vi "why_jiggle.vi"() -> ()   [LabVIEW 2023]
uses:
  Supporting VIs/Sampling frequency.ctl
  Arun_test/Control 1.ctl
  Supporting VIs/Logic states.ctl
  Supporting VIs/Motor states.ctl
  Supporting VIs/Queue names.ctl
  <instrlib>/Arcus Driver 3.0.0/ArcusUsbComm/classes/Controller/_Controller.lvclass
  <instrlib>/Arcus Driver 3.0.0/ArcusUsbComm/common/controls/linear_direction.ctl
  Supporting VIs/Axes indices.ctl
  <vilib>/DAQmx/read.llb/DAQmx Read (Analog 1D DBL NChan 1Samp).vi
  <vilib>/Analysis/baseanly.llb/Vector x A.vi
  <vilib>/Analysis/baseanly.llb/A x Vector.vi
  <vilib>/DAQmx/create/channels.llb/DAQmx Create Channel (AI-Voltage-Basic).vi
  <vilib>/DAQmx/configure/timing.llb/DAQmx Timing (Sample Clock).vi
  <vilib>/DAQmx/miscellaneous.llb/DAQmx Fill In Error Info.vi
  <vilib>/Utility/file.llb/Write Delimited Spreadsheet (string).vi
  <vilib>/addons/control/pid/pid.llb/PID (DBL).vi
  <vilib>/Utility/file.llb/Write Delimited Spreadsheet (DBL).vi
  <vilib>/Analysis/NI_AALBase.lvlib
  <instrlib>/Arcus Driver 3.0.0/ArcusUsbComm/libraries/common.lvlib
  <vilib>/addons/control/pid/NI_PID_pid.lvlib
panel:
  in  "Wait [min]":dbl=30.0 format="%.2g"
  in  "Wait ?":bool=TRUE
  in  "Save file name":path=path "C:/Users/Egberts/Desktop/Tribometer/August 2020 Measurements/Tribometer/Late August 2020/test.txt"
  out "Apprx. Min Left":i32
  out "Cycles left":i32
  out "Test Progress":i32(slide) scale=0.0..5999.0
  in  "PID gains":T1={"proportional gain (Kc)"=0.02, "integral time (Ti, min)"=0.1, "derivative time (Td, min)"=0.001} {"derivative time (Td, min)" format="%.3f"; "integral time (Ti, min)" format="%.3f"; "proportional gain (Kc)" format="%.3f"}
  in  "output range":cluster{"output high":dbl, "output low":dbl}={"output high"=2.0, "output low"=-2.0} {"output low" format="%.2f"; "output high" format="%.2f"}
  out "x-position":i32
  out "z-position":string
  in  "set zero":bool
  out "Correction loop":i32
  out "received P":i32
  out "Actual Load":dbl
  out "Correction [N]":dbl format="%.2f"
  out "correction [p]":dbl
  out "to PID":i32
  out "dt out (s)":dbl=0.25 format="%.3f"
  in  "Testing Load [N]":dbl=20.0
  in  "Wear cycles":i32=3000
  in  "Track length [mm]":i32=15
  in  "x-Velocity [mm/s]":i32=6
  out "Manual control":bool
  in  "Approach":bool
  in  "DAQmx Device Name":tag="Dev1"
  in  "Out":bool
  in  "In":bool
  in  "Left":bool
  in  "Right":bool
  in  "Up":bool
  out "Estimated friction coefficient":dbl(graph)=-0.11599973982411911
  out "Smooth x":dbl(graph)=-1.1532615270996815
  out "Smooth z":dbl(graph)=9.94193201509139
  out "Dequeued Data":dbl[](graph)=[9.378691263157721, 10.717600289594278, 8.438969804942502, 9.318124790458075, 8.681089909963866, 9.970529667476073, 10.834102440336615, 9.183821958337319, 9.334582664259113, 9.226213467034226, 10.238553338370796, 11.173780758664948, 8.690449558950064, 9.261606371512476, 8.790570665988898, 9.887706352746802, 11.038667014275244, 8.916330650848511, 9.104119720861869, 8.923720573303449]
  out "Fixed amplitude Load":T2=8.923720573303449
  in  "ABORT":bool
  in  "Down":bool
  out "Aborted":bool
  out "Mean z":dbl[](array[numeric])
  out "Current reading":dbl[](array[numeric])
  in  "Averaging Level":i32=12
  out "Mean x":dbl[](array[numeric])
  out "Completed":bool
  out "Testing":bool
  out "Approaching":bool
  in  "TARE":bool
  in  "Sampling frequency (rate)":T3=100 items=["1000 Hz"=1000, " 500 Hz"=500, " 250 Hz"=250, "100 Hz"=100, "50 Hz"=50, "10 Hz"=10, "1 Hz"=1]
  in  "Calibration file":path=path "C:/Users/Egberts/Desktop/ATI Industrial Automation/FT21774.cal"
  # "Originally used to measure \nthe amount of positions needed\nto perform fast approach"
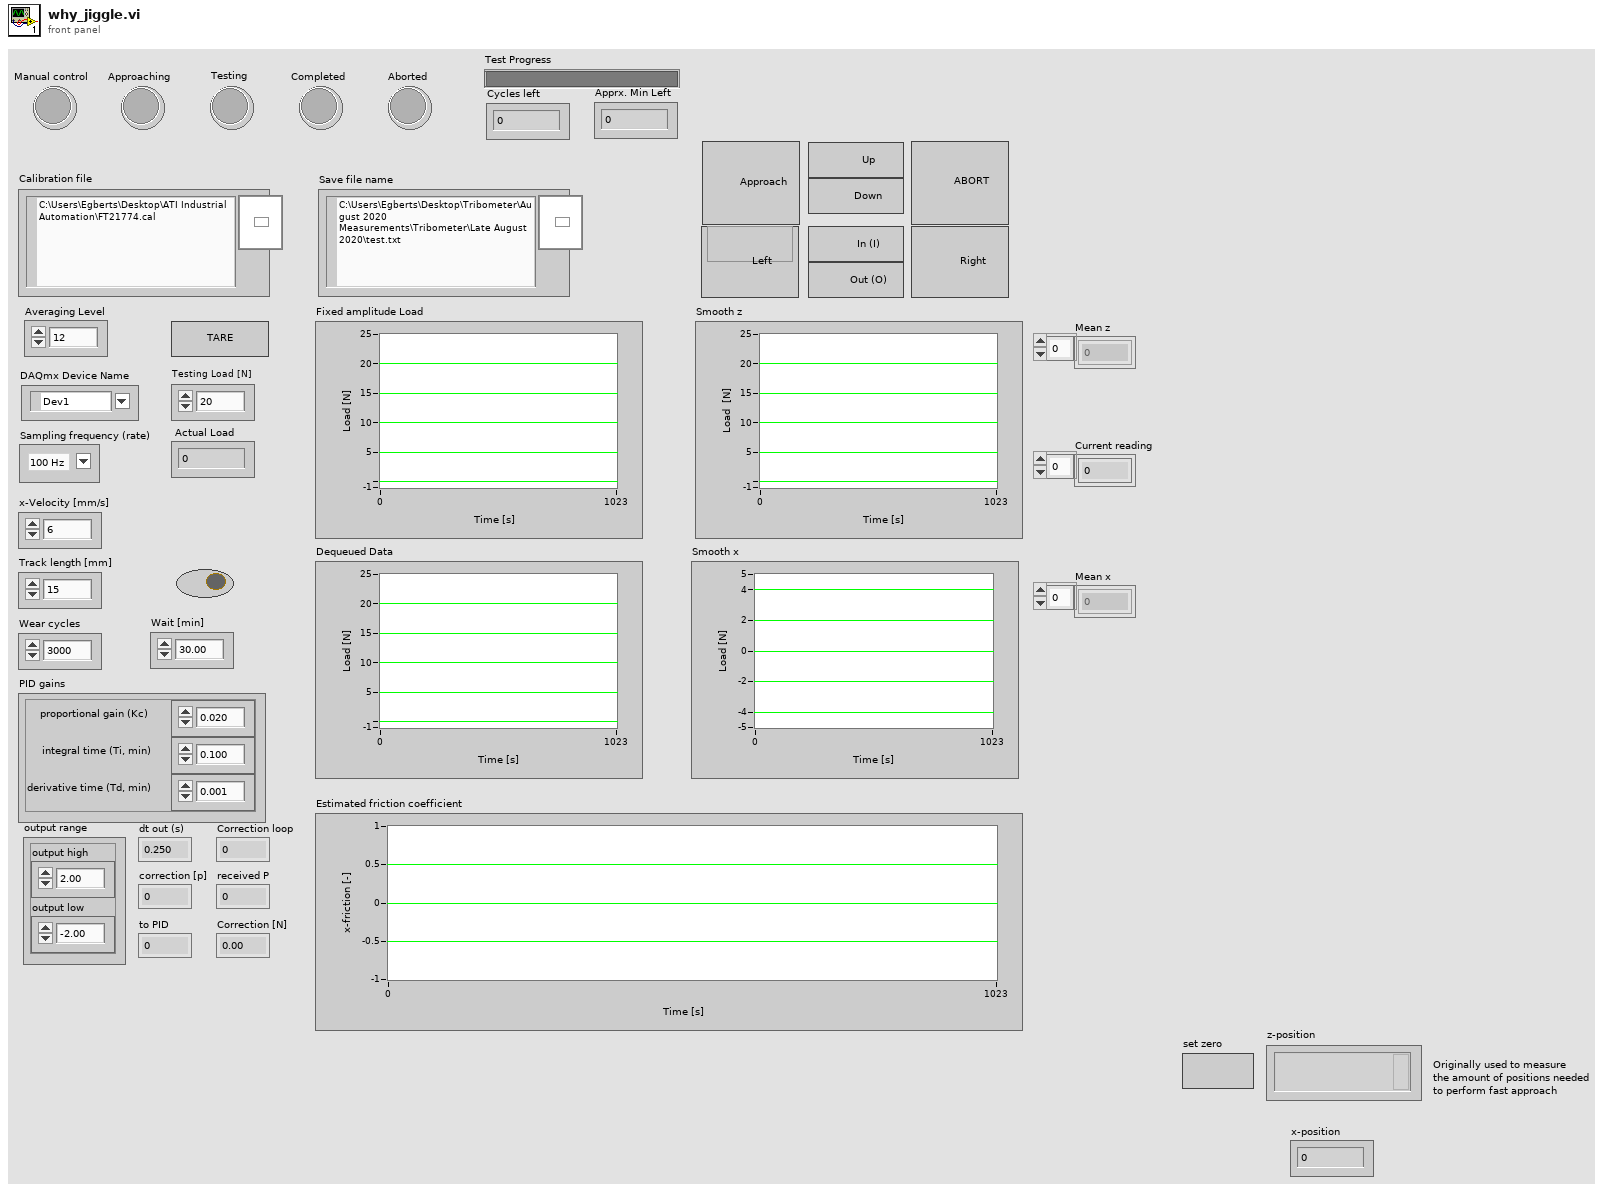
[diagram p1: front panel]
types:
  T1 = cluster{"proportional gain (Kc)":dbl, "integral time (Ti, min)":dbl, "derivative time (Td, min)":dbl}
  T2 = typedef "Control 1.ctl" = dbl
  T3 = typedef "Sampling frequency.ctl" = u16
  T4 = typedef "Queue names.ctl" = enum16{"Cell queue name", "z-axis ref queue", "x-axis ref queue", "tangent-axis ref queue", "y-axis ref queue", "to PID", "Feedback"}
  T5 = typedef "Motor states.ctl" = enum16{"Initialize", "Manual control", "Approaching", "Testing", "Terminate"}
  T6 = typedef "Logic states.ctl" = enum16{"Initialize", "Process", "Terminate"}
  T7 = enum8{"Enabled", "Disabled", "Disabled and Grayed Out"}
  T8 = cluster{"queue out":refnum<queue>, "error out":errorcluster}
  T9 = cluster{"task out":refnum<k21>, "error out":errorcluster}
  T10 = cluster{"reference (out)":refnum<class "_Controller.lvclass">, "error out":errorcluster}
  T11 = typedef "Axes indices.ctl" = enum16{"y-axis", "x-axis", "z-axis"}
  T12 = cluster{"queue out":refnum<queue>, "queue out":refnum<queue>, "queue out":refnum<queue>}
  T13 = typedef "common.lvlib/linear_direction.ctl" = enum16{"POS (+)", "NEG (-)"}
  T14 = typedef "lveventtype.ctl" = enum32{"Null", "Timeout", "Annotation Menu Selection", "Annotation Menu Selection?", "App Instance Close", "App Instance Close?", "Autoscale Range Change", "Bookmark Info Change", "Cell Edit", "Cell Edit?", "Cursor Grab", "Cursor Grab?", "Cursor Menu Selection", "Cursor Menu Selection?", "Cursor Move", "Cursor Release", "Data Change", "Direction Change", "Display State Change", "Drag Ended", "Drag Enter", "Drag Leave", "Drag Over", "Drag Source Update", "Drag Starting", "Drag Starting?", "Drop", "Exec State Change", "Key Down", "Key Down?", "Key Repeat", "Key Repeat?", "Key Up", "Listbox Double Click", "Menu Activation?", "Menu Selection (App)", "Menu Selection? (App)", "Menu Selection (User)", "Mouse Down", "Mouse Down?", "Mouse Enter", "Mouse Leave", "Mouse Move", "Mouse Up", "Mouse Wheel", "NI Security User Change (App)", "Pane Size", "Panel Close", "Panel Close?", "Panel Resize", "Plot Attribute Change", "Scale Range Change", "Shortcut Menu Activation?", "Shortcut Menu Selection (App)", "Shortcut Menu Selection? (App)", "Shortcut Menu Selection (User)", "Tree Double Click", "Tree Drag", "Tree Drag?", "Tree Drop", "Tree Drop?", "Tree Item Close", "Tree Item Close?", "Tree Item Open", "Tree Item Open?", "User Event", "Value Change"}
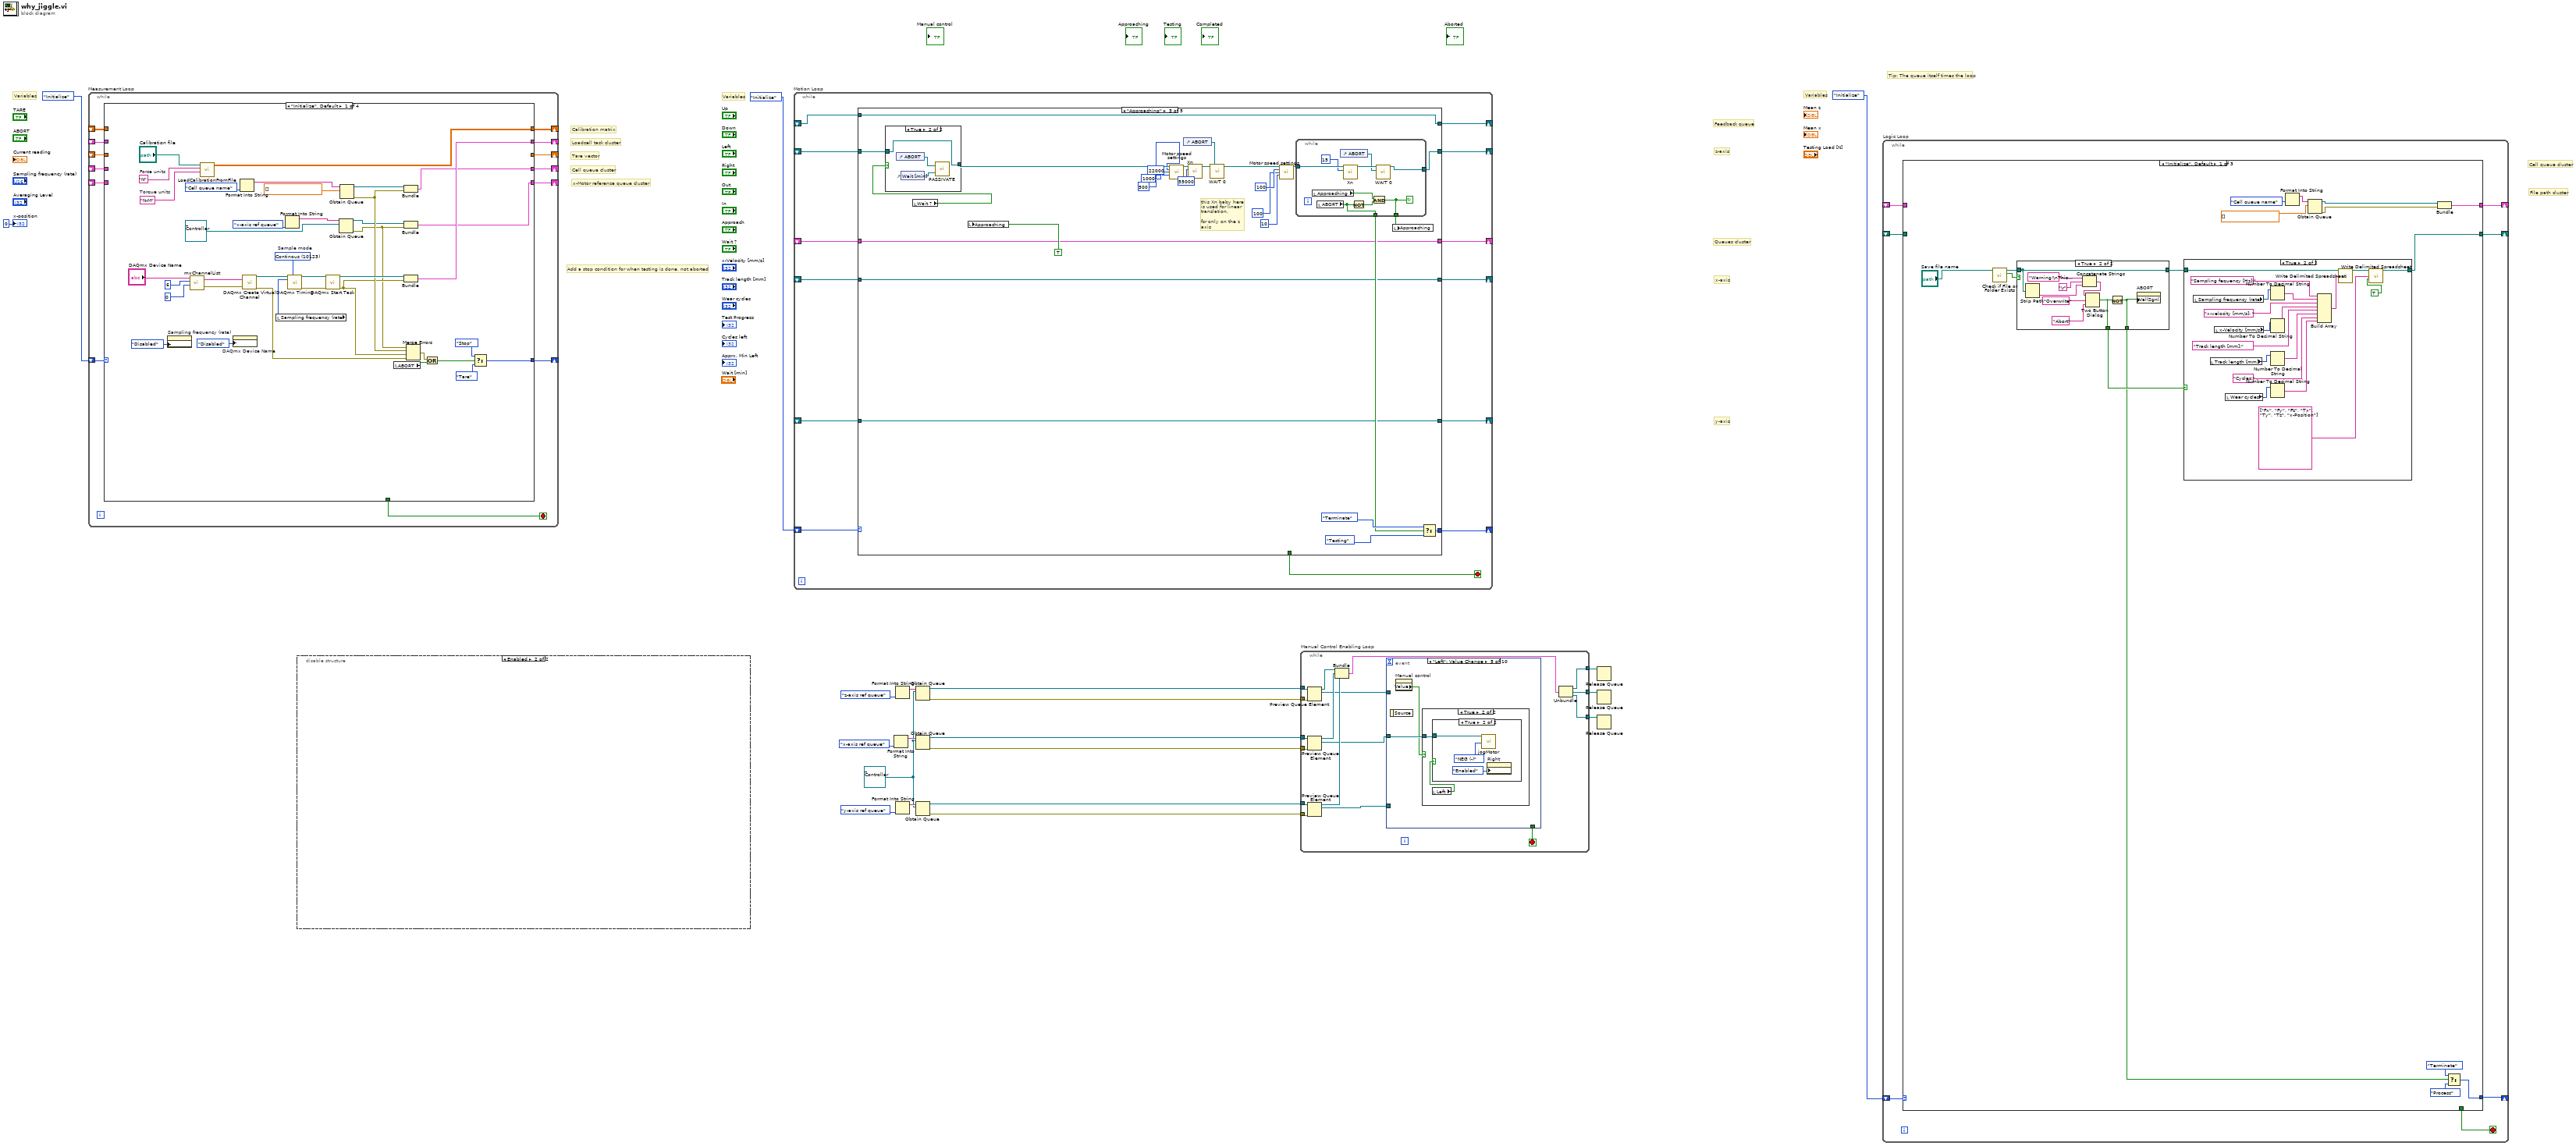
[diagram p0: block diagram]
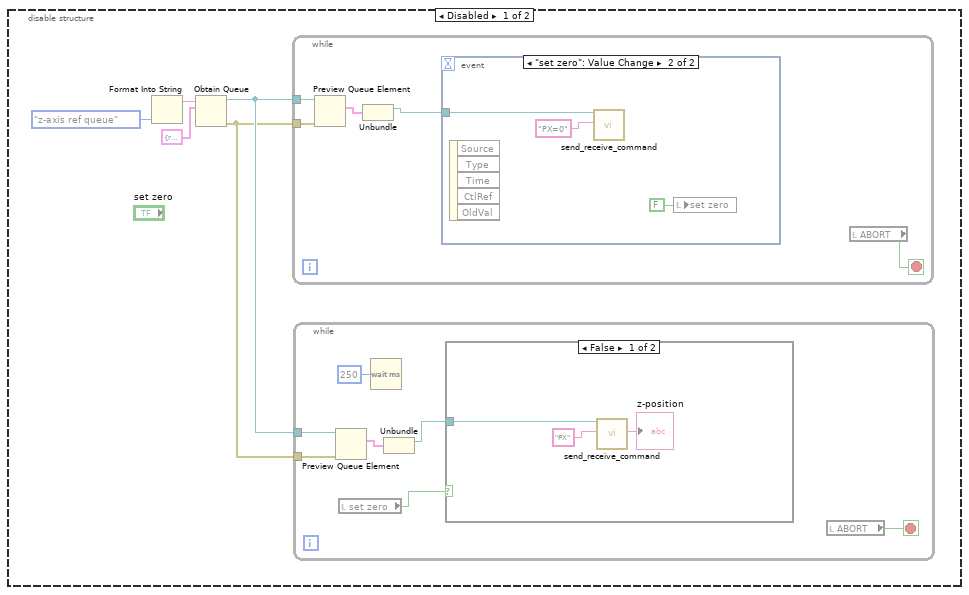
[diagram p2: hidden frame]
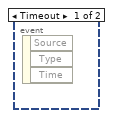
[diagram p4: hidden frame]
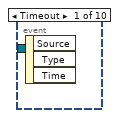
[diagram p5: hidden frame]
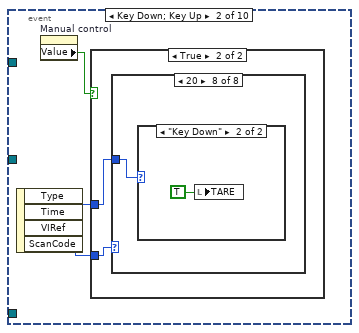
[diagram p6: hidden frame]
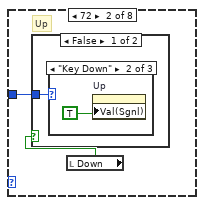
[diagram p9: hidden frame]
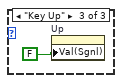
[diagram p11: hidden frame]
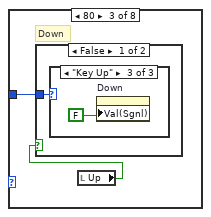
[diagram p13: hidden frame]
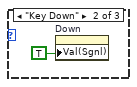
[diagram p15: hidden frame]
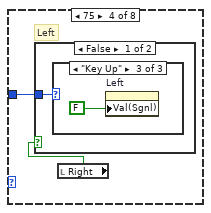
[diagram p17: hidden frame]
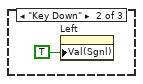
[diagram p19: hidden frame]
diagram:
  w1 = refnum<class "_Controller.lvclass"> refnum ("Controller in")
  # "Feedback queue"
  # "Queues cluster"
  # "x-Motor reference queue cluster"
  # "Add a stop condition for when testing is done, not aborted"
  # "y-axis"
  # "x-axis"
  # "z-axis"
  # "Variables"
  # "Variables"
  # "File path cluster"
  # "Cell queue cluster"
  # "Tip: The queue itself times the loop"
  # "Variables"
  # "Cell queue cluster"
  # "Loadcell task cluster"
  # "Tare vector"
  # "Calibration matrix"
  n1 = while "Measurement Loop" {
    shift-right: [w32] -> _
    shift-left: enum16{"Initialize", "Tare", "Measure", "Stop"}."Initialize" ("Enum") -> [w33]
    shift-right: [w27] -> _
    shift-left: _ -> [w26]
    shift-right: [w31] -> _
    shift-left: _ -> [w29]
    shift-right: [w30] -> _
    shift-left: _ -> [w28]
    shift-right: [w23] -> _
    shift-left: _ -> [w24]
    shift-right: [w22] -> _
    shift-left: _ -> [w21]
    stop <- w25 stop-if-true
    n2 = case shown="\"Initialize\", Default" w33 {
      tunnel: [w55 w80 w115 _] -> w32
      tunnel: [_ w87 _ _] -> w31
      tunnel: [w59 w79 w117 _] -> w30
      tunnel: w28 -> [_ w79 w117 w182]
      tunnel: w29 -> [_ _ w118 _]
      tunnel: [w58 w86 w116 _] -> w27
      tunnel: w26 -> [_ w86 w116 _]
      tunnel: [_ _ _ TRUE] -> w25
      tunnel: w24 -> [_ w74 w103 w179]
      tunnel: [w50 w74 w104 _] -> w23
      tunnel: [w39 w72 w111 _] -> w22
      tunnel: w21 -> [_ w72 w111 w173]
      frame "Initialize", Default {
        w63 = u16 10123 items=["Continous"=10123, "Finite"=10178, "Hardware Timed"=12522]  # Sample mode
        w70 = "N-M"  # Torque units
        w69 = "N"  # Force units
        n3 = property on="Sampling frequency (rate)" class="Ring (strict)"("DisabledEnum"=T7."Disabled" ("Disabled")) -> ()  [unwired: 2 in, 2 out]
        n4 = call "mxChannelList.vi"("First Channel"=0, "Number of Channels"=6, "DAQmx Device Name"="DAQmx Device Name") -> ("error out"=w65:errorcluster, "Channel List"=w66:string)  [unwired: 1 in]
        n5 = call "LoadCalibrationFromFile.vi"("User Torque Units"=w70, "User Force Units"=w69, "Cal File Path"="Calibration file") -> ("Calibration Matrix"=w58:dbl[][])  [unwired: 1 in, 3 out]
        n6 = property on="DAQmx Device Name" class="DAQmxName"("DisabledEnum"=T7."Disabled" ("Disabled")) -> ()  [unwired: 2 in, 2 out]
        n7 = Format Into String(Queue_names."Cell queue name" ("Enum")) -> (resulting string=w37:string)  [unwired: 3 in, 1 out]
        n8 = call-poly <vilib>:"DAQmx Create Virtual Channel.vi"("physical channels"=w66, "error in"=w65) -> ("task out"=w64:refnum<k21>, "error out"=w43:errorcluster)  [unwired: 12 in]
        n9 = local read "Sampling frequency (rate)"() -> (w49:T3)
        n10 = Format Into String(Queue_names."x-axis ref queue" ("Enum")) -> (resulting string=w35:string)  [unwired: 3 in, 1 out]
        n11 = call-poly <vilib>:"DAQmx Timing.vi"("task/channels in"=w64, "sample mode"=w63, "rate"=w49) -> ("task out"=w62:refnum<k21>, "error out"=w61:errorcluster)  [unwired: 11 in]
        n12 = call <vilib>:"DAQmx Start Task.vi"("task/channels in"=w62, "error in"=w61) -> ("task out"=w60:refnum<k21>, "error out"=w44:errorcluster)  [unwired: 12 in]
        n13 = Obtain Queue(name (unnamed)=w35, element data type=refnum<class "_Controller.lvclass"> refnum ("reference (in)")) -> (queue out=w41:refnum<queue>, error out=w40:errorcluster)  [unwired: 3 in, 1 out]
        n14 = Obtain Queue(name (unnamed)=w37, element data type=dbl[] []) -> (queue out=w51:refnum<queue>, error out=w45:errorcluster)  [unwired: 3 in, 1 out]
        n15 = local read "ABORT"() -> (w53:bool)
        n16 = Bundle("queue out"=w51, "error out"=w45) -> (w50:T8)  [unwired: 1 in]
        n17 = Bundle("queue out"=w41, "error out"=w40) -> (w39:T8)  [unwired: 1 in]
        n18 = Bundle("task out"=w60, "error out"=w44) -> (w59:T9)  [unwired: 1 in]
        n19 = Merge Errors(w40, w45, w44, w43) -> (w42:errorcluster)
        n20 = Compound Arithmetic op=OR(w42, w53) -> (w54:bool)
        n21 = Select(t=enum16{"Initialize", "Tare", "Measure", "Stop"}."Stop" ("Enum"), s=w54, f=enum16{"Initialize", "Tare", "Measure", "Stop"}."Tare" ("Enum")) -> (s? t:f=w55:enum16{"Initialize", "Tare", "Measure", "Stop"})
      }
      frame "Tare" {
        n22 = local read "Averaging Level"() -> (w73:i32)
        n23 = for {
          N: w73 -> [_]
          tunnel: w79 -> [w93]
          shift-right: [w95] -> w77
          shift-left: dbl[][] [] -> [w94]
          tunnel: [w92] -> w76
          tunnel: [FALSE] -> w75
          n24 = Unbundle(w93) -> ("task out"=w98:refnum<k21>, "error out"=w97:errorcluster)
          n25 = call-poly <vilib>:"DAQmx Read.vi"("task/channels in"=w98, "error in"=w97) -> ("data"=w96:dbl[], "error out"=w92:errorcluster)  [unwired: 11 in, 1 out]
          n26 = Build Array (concatenate)(w94, w96) -> (w95:dbl[][])
        }
        n27 = local write "TARE"(w75) -> ()
        n28 = Matrix Size(0:w77) -> (1:w88:i32)  [unwired: 1 out]
        n29 = Reciprocal(x=w88) -> (1/x=w89:dbl)
        n30 = Unbundle By Name(w76) -> ("status"=w81:bool)
        n31 = local read "ABORT"() -> (w82:bool)
        n32 = Initialize Array(w89, w88) -> (w90:dbl[])
        n33 = Or(x=w81, y=w82) -> (x .or. y?=w85:bool)
        n34 = call-poly <vilib>:"A x B.vi"("Matrix A"=w77, "Vector V'"=w90) -> ("V' x A"=w87:dbl[])  [unwired: 1 out]
        n35 = Select(t=enum16{"Initialize", "Tare", "Measure", "Stop"}."Stop" ("Enum"), s=w85, f=enum16{"Initialize", "Tare", "Measure", "Stop"}."Measure" ("Enum")) -> (s? t:f=w80:enum16{"Initialize", "Tare", "Measure", "Stop"})
      }
      frame "Measure" {
        n36 = Unbundle(w111) -> ("queue out"=w100:refnum<queue>, "error out"=w99:errorcluster)
        n37 = Unbundle(w103) -> ("queue out"=w102:refnum<queue>, "error out"=w101:errorcluster)
        n38 = Unbundle(w111) -> ("queue out"=w110:refnum<queue>, "error out"=w109:errorcluster)
        n39 = Unbundle(w117) -> ("task out"=w108:refnum<k21>, "error out"=w107:errorcluster)
        n40 = while {
          tunnel: w118 -> [w159]
          tunnel: w116 -> [w151]
          tunnel: [w149] -> w112
          tunnel: w110 -> [w141]
          tunnel: w109 -> [w140]
          tunnel: w108 -> [w139]
          tunnel: w107 -> [w138]
          tunnel: [w137] -> w106
          tunnel: [w136] -> w105
          tunnel: w102 -> [w135]
          tunnel: w101 -> [w134]
          stop <- w154 stop-if-true
          w156 = u16 2 items=["x-load", "y-load", "z-load", "x-torque", "y-torque", "z-torque"]
          n41 = Get Queue Status(queue=w141, error in (no error)=w140) -> (# elements in queue=w145:i32)  [unwired: 1 in, 7 out]
          n42 = local read "Testing"() -> (w144:bool)
          n43 = call-poly <vilib>:"DAQmx Read.vi"("task/channels in"=w139, "error in"=w138) -> ("data"=w152:dbl[], "error out"=w150:errorcluster)  [unwired: 11 in, 1 out]
          n44 = Not Equal To 0?(x=w145) -> (x != 0?=w143:bool)
          n45 = And(x=w143, y=w144) -> (x .and. y?=w142:bool)
          n46 = Subtract(x=w152, y=w159) -> (x-y=w158:dbl[])
          n47 = call-poly <vilib>:"A x B.vi"("Vector"=w158, "A"=w151) -> ("A x Vector"=w147:dbl[])  [unwired: 1 out]
          n48 = case shown="True" w142 {
            tunnel: [FALSE ("status") w170] -> w148
            tunnel: w147 -> [_ w169]
            tunnel: w135 -> [w161 w166]
            tunnel: w134 -> [w160 w165]
            tunnel: [w161 w164] -> w137
            tunnel: [w160 w163] -> w136
            frame False {
            }
            frame True {
              n49 = local read "x-position"() -> (w167:i32)
              n50 = Build Array (concatenate)(w169, w167) -> (w168:dbl[])
              n51 = Enqueue Element(queue=w166, element=w168, error in (no error)=w165) -> (queue out=w164:refnum<queue>, error out=w163:errorcluster)  [unwired: 1 in, 1 out]
              n52 = Unbundle By Name(w163) -> ("status"=w170:bool)
            }
          }
          n53 = local write "Current reading"(w147) -> ()
          n54 = Index Array(array=w147, index=w156) -> (element=w157:dbl)
          n55 = Negate(x=w157) -> (-x=→"Fixed amplitude Load":dbl)
          n56 = local read "TARE"() -> (w149:bool)
          n57 = Unbundle By Name(w150) -> ("status"=w153:bool)
          n58 = local read "ABORT"() -> (w155:bool)
          n59 = Compound Arithmetic op=OR(w148, w149, w155, w153) -> (w154:bool)
        }
        n60 = while {
          tunnel: w100 -> [w120]
          tunnel: w99 -> [w119]
          stop <- w122 stop-if-true
          n61 = local read "Testing"() -> (w126:bool)
          n62 = Get Queue Status(queue=w120, error in (no error)=w119) -> (queue out=w124:refnum<queue>, # elements in queue=w128:i32)  [unwired: 1 in, 6 out]
          n63 = Not Equal To 0?(x=w128) -> (x != 0?=w127:bool)
          n64 = And(x=w127, y=w126) -> (x .and. y?=w125:bool)
          n65 = case shown="True" w125 {
            tunnel: w124 -> [_ w130]
            frame False {
            }
            frame True {
              n66 = Preview Queue Element(queue=w130) -> (element=w129:refnum<class "_Controller.lvclass">)  [unwired: 2 in, 3 out]
              n67 = call <instrlib>:"send_receive_command.vi"("reference (in)"=w129, "ASCII Command (in)"="PX") -> ("response (out)"=w132:string)  [unwired: 13 in, 4 out]
              n68 = Decimal String To Number(string=w132) -> (number=w131:i32)  [unwired: 2 in, 1 out]
              n69 = local write "x-position"(w131) -> ()
            }
          }
          n70 = local read "ABORT"() -> (w123:bool)
          n71 = local read "TARE"() -> (w121:bool)
          n72 = Or(x=w123, y=w121) -> (x .or. y?=w122:bool)
        }
        n73 = Select(t=enum16{"Initialize", "Tare", "Measure", "Stop"}."Tare" ("Enum"), s=w112, f=enum16{"Initialize", "Tare", "Measure", "Stop"}."Stop" ("Enum")) -> (s? t:f=w115:enum16{"Initialize", "Tare", "Measure", "Stop"})
        n74 = Bundle("queue out"=w106, "error out"=w105) -> (w104:T8)  [unwired: 1 in]
      }
      frame "Stop" {
        n75 = Unbundle(w182) -> ("task out"=w181:refnum<k21>, "error out"=w180:errorcluster)
        n76 = Unbundle(w179) -> ("queue out"=w178:refnum<queue>, "error out"=w177:errorcluster)
        n77 = Unbundle(w173) -> ("queue out"=w172:refnum<queue>, "error out"=w171:errorcluster)
        n78 = call <vilib>:"DAQmx Clear Task.vi"("task in"=w181, "error in"=w180) -> ()  [unwired: 13 in, 1 out]
        n79 = Release Queue(queue=w172, error in (no error)=w171) -> ()  [unwired: 1 in, 3 out]
        n80 = Release Queue(queue=w178, force destroy? (F)=FALSE, error in (no error)=w177) -> ()  [unwired: 3 out]
        n81 = property on="Sampling frequency (rate)" class="Ring (strict)"("DisabledEnum"=T7."Enabled" ("Disabled")) -> ()  [unwired: 2 in, 2 out]
        n82 = property on="DAQmx Device Name" class="DAQmxName"("DisabledEnum"=T7."Disabled" ("Disabled")) -> ()  [unwired: 2 in, 2 out]
      }
    }
  }
  n83 = disable-structure shown="Enabled" {
    frame Disabled {
      n84 = Format Into String(Queue_names."z-axis ref queue" ("Enum")) -> (resulting string=w187:string)  [unwired: 3 in, 1 out]
      n85 = Obtain Queue(name (unnamed)=w187, element data type=T10 {"reference (out)"=refnum, "error out"={"status"=FALSE, "code"=0, "source"=""}} ("output cluster")) -> (queue out=w185:refnum<queue>, error out=w184:errorcluster)  [unwired: 3 in, 1 out]
      n86 = while {
        tunnel: w185 -> [w203]
        tunnel: w184 -> [w202]
        stop <- w199 stop-if-true
        n87 = Preview Queue Element(queue=w203, error in (no error)=w202) -> (element=w201:T10)  [unwired: 1 in, 3 out]
        n88 = Unbundle(w201) -> ("reference (out)"=w200:refnum<class "_Controller.lvclass">)  [unwired: 1 out]
        n89 = event shown="[1] \"set zero\": Value Change" {
          selector: _ -> [_ _]
          dyn-events: _ -> [_ _]
          timeout: _ -> [_ _]
          tunnel: w200 -> [_ w206]
          event Timeout {
            n90 = event-data() -> ()  [unwired: 1 in, 3 out]
          }
          event "set zero": Value Change {
            n91 = event-data() -> ()  [unwired: 1 in, 5 out]
            n92 = call <instrlib>:"send_receive_command.vi"("reference (in)"=w206, "ASCII Command (in)"="PX=0") -> ()  [unwired: 13 in, 5 out]
            n93 = local write "set zero"(FALSE ("set zero")) -> ()
          }
        }
        n94 = local read "ABORT"() -> (w199:bool)
      }
      n95 = while {
        tunnel: w185 -> [w192]
        tunnel: w184 -> [w191]
        stop <- w194 stop-if-true
        n96 = Preview Queue Element(queue=w192, error in (no error)=w191) -> (element=w193:T10)  [unwired: 1 in, 3 out]
        n97 = local read "set zero"() -> (w189:bool)
        n98 = Wait (ms)(milliseconds to wait=u32 250) -> ()  [unwired: 1 out]
        n99 = Unbundle(w193) -> ("reference (out)"=w190:refnum<class "_Controller.lvclass">)  [unwired: 1 out]
        n100 = case shown="False" w189 {
          tunnel: w190 -> [w197 _]
          frame False {
            n101 = call <instrlib>:"send_receive_command.vi"("reference (in)"=w197, "ASCII Command (in)"="PX") -> ("response (out)"=→"z-position":string)  [unwired: 13 in, 4 out]
          }
          frame True {
          }
        }
        n102 = local read "ABORT"() -> (w194:bool)
      }
    }
    frame Enabled {
    }
  }
  n103 = while "Motion Loop" {
    shift-right: [w218] -> _
    shift-left: Motor_states."Initialize" -> [w219]
    shift-right: [w209] -> _
    shift-left: _ -> [w217]
    shift-right: [w208] -> _
    shift-left: _ -> [w216]
    shift-right: [w207] -> _
    shift-left: _ -> [w215]
    shift-right: [w213] -> _
    shift-left: _ -> [w212]
    shift-right: [w211] -> _
    shift-left: _ -> [w210]
    stop <- w214 stop-if-true
    n104 = case shown="\"Approaching\"" w219 {
      tunnel: [Motor_states."Manual control" w281 w313 Motor_states."Terminate" _] -> w218
      tunnel: w217 -> [_ w266 w297 w335 w401]
      tunnel: w216 -> [_ w264 w301 w333 w400]
      tunnel: w215 -> [_ w262 w300 w331 w399]
      tunnel: [_ _ _ _ w407] -> w214
      tunnel: [w231 w268 w305 w344 _] -> w213
      tunnel: w212 -> [_ w268 w305 w344 w406]
      tunnel: [w226 w267 w304 w343 _] -> w211
      tunnel: w210 -> [_ w267 w304 w343 w402]
      tunnel: [w225 w265 w302 w334 _] -> w209
      tunnel: [w224 w263 w301 w332 _] -> w208
      tunnel: [w223 w261 w300 w331 _] -> w207
      frame "Initialize" {
        w220 = TRUE
        w222 = FALSE ("Approach")
        n105 = local write "Test Progress"(0 ("Test Progress")) -> ()
        n106 = local write "Testing"(w222) -> ()
        n107 = local write "Aborted"(w222) -> ()
        n108 = local write "Approach"(w222) -> ()
        n109 = local write "Approaching"(w222) -> ()
        n110 = local write "Completed"(w222) -> ()
        n111 = call <instrlib>:"initialize.vi"("device_index (in) [0=def]"=Axes_indices."z-axis", "clear_buffer? (T)"=w220) -> ("reference (out)"=w256:refnum<class "_Controller.lvclass">)  [unwired: 16 in, 1 out]
        n112 = call <instrlib>:"initialize.vi"("device_index (in) [0=def]"=Axes_indices."x-axis", "clear_buffer? (T)"=w220) -> ("reference (out)"=w255:refnum<class "_Controller.lvclass">)  [unwired: 16 in, 1 out]
        n113 = call <instrlib>:"initialize.vi"("device_index (in) [0=def]"=Axes_indices."y-axis", "clear_buffer? (T)"=w220) -> ("reference (out)"=w254:refnum<class "_Controller.lvclass">)  [unwired: 16 in, 1 out]
        n114 = call <instrlib>:"send_receive_command.vi"("reference (in)"=w256, "ASCII Command (in)"="SR0=0") -> ("reference (out)"=w248:refnum<class "_Controller.lvclass">)  [unwired: 13 in, 4 out]
        n115 = call <instrlib>:"send_receive_command.vi"("reference (in)"=w255, "ASCII Command (in)"="SR0=0") -> ("reference (out)"=w249:refnum<class "_Controller.lvclass">)  [unwired: 13 in, 4 out]
        n116 = call <instrlib>:"send_receive_command.vi"("reference (in)"=w254, "ASCII Command (in)"="SR0=0") -> ("reference (out)"=w250:refnum<class "_Controller.lvclass">)  [unwired: 13 in, 4 out]
        n117 = call <instrlib>:"send_receive_command.vi"("reference (in)"=w248, "ASCII Command (in)"="INC") -> ("reference (out)"=w225:refnum<class "_Controller.lvclass">)  [unwired: 13 in, 4 out]
        n118 = call <instrlib>:"send_receive_command.vi"("reference (in)"=w249, "ASCII Command (in)"="INC") -> ("reference (out)"=w224:refnum<class "_Controller.lvclass">)  [unwired: 13 in, 4 out]
        n119 = call <instrlib>:"send_receive_command.vi"("reference (in)"=w250, "ASCII Command (in)"="INC") -> ("reference (out)"=w223:refnum<class "_Controller.lvclass">)  [unwired: 13 in, 4 out]
        n120 = Format Into String(Queue_names."Feedback" ("Enum")) -> (resulting string=w230:string)  [unwired: 3 in, 1 out]
        n121 = Format Into String(Queue_names."x-axis ref queue" ("Enum")) -> (resulting string=w239:string)  [unwired: 3 in, 1 out]
        n122 = Format Into String(Queue_names."z-axis ref queue" ("Enum")) -> (resulting string=w240:string)  [unwired: 3 in, 1 out]
        n123 = Obtain Queue(max queue size (-1, unlimited)=1, name (unnamed)=w230, element data type=0) -> (queue out=w226:refnum<queue>)  [unwired: 2 in, 2 out]
        n124 = Format Into String(Queue_names."y-axis ref queue" ("Enum")) -> (resulting string=w238:string)  [unwired: 3 in, 1 out]
        n125 = Obtain Queue(name (unnamed)=w240, element data type=w225) -> (queue out=w247:refnum<queue>)  [unwired: 3 in, 2 out]
        n126 = Obtain Queue(name (unnamed)=w239, element data type=w224) -> (queue out=w246:refnum<queue>)  [unwired: 3 in, 2 out]
        n127 = Obtain Queue(name (unnamed)=w238, element data type=w223) -> (queue out=w245:refnum<queue>, error out=w244:errorcluster)  [unwired: 3 in, 1 out]
        n128 = Enqueue Element(queue=w247, element=w225) -> (queue out=w234:refnum<queue>)  [unwired: 2 in, 2 out]
        n129 = Enqueue Element(queue=w246, element=w224) -> (queue out=w233:refnum<queue>)  [unwired: 2 in, 2 out]
        n130 = Enqueue Element(queue=w245, element=w223, error in (no error)=w244) -> (queue out=w232:refnum<queue>)  [unwired: 1 in, 2 out]
        n131 = Bundle("queue out"=w234, "queue out"=w233, "queue out"=w232) -> (w231:T12)  [unwired: 1 in]
      }
      frame "Manual control" {
        n132 = local write "Manual control"(TRUE ("Manual control")) -> ()
        n133 = call "Motor speed settings.vi"("reference (in)"=w266, "HSPD"=13000 ("High Speed"), "LSPD"=100 ("Low Speed"), "ACC"=250 ("Acceleration Time")) -> ("reference (out)"=w265:refnum<class "_Controller.lvclass">)  [unwired: 10 in, 1 out]
        n134 = call "Motor speed settings.vi"("reference (in)"=w264, "HSPD"=13000 ("High Speed"), "LSPD"=100 ("Low Speed"), "ACC"=250 ("Acceleration Time")) -> ("reference (out)"=w263:refnum<class "_Controller.lvclass">)  [unwired: 10 in, 1 out]
        n135 = call "Motor speed settings.vi"("reference (in)"=w262, "HSPD"=13000 ("High Speed"), "LSPD"=100 ("Low Speed"), "ACC"=250 ("Acceleration Time")) -> ("reference (out)"=w261:refnum<class "_Controller.lvclass">)  [unwired: 10 in, 1 out]
        n136 = while {
          tunnel: [w287] -> w270
          stop <- w286 stop-if-true
          n137 = Wait Until Next ms Multiple(millisecond multiple=u32 150) -> ()  [unwired: 1 out]
          n138 = local read "Approach"() -> (w288:bool)
          n139 = local read "ABORT"() -> (w287:bool)
          n140 = Or(x=w288, y=w287) -> (x .or. y?=w286:bool)
        }
        n141 = case shown="False" w270 {
          tunnel: [FALSE TRUE] -> w269
          frame False {
          }
          frame True {
          }
        }
        n142 = local write "Manual control"(w269) -> ()
        n143 = Select(t=Motor_states."Terminate", s=w270, f=Motor_states."Approaching") -> (s? t:f=w281:T5)
      }
      frame "Approaching" {
        # "this Xn baby here \nis used for linear\ntranslation.\n\nfsr only on the z axis"
        n144 = local read "Wait ?"() -> (w299:bool)
        n145 = case shown="True" w299 {
          tunnel: [w316 w319] -> w298
          tunnel: w297 -> [w316 w319]
          frame False {
          }
          frame True {
            n146 = control-ref of="ABORT"() -> (w318:refnum<vi>)
            n147 = control-ref of="Wait [min]"() -> (w317:refnum<vi>)
            n148 = call "PASSIVATE.vi"("reference"=w317, "Boolean in"=w318) -> ()  [unwired: 1 in]
          }
        }
        n149 = local write "Approaching"(TRUE ("Approaching")) -> ()
        n150 = call "Motor speed settings.vi"("reference (in)"=w298, "HSPD"=22000 ("High Speed"), "LSPD"=1000 ("Low Speed"), "ACC"=500 ("Acceleration Time")) -> ("reference (out)"=w292:refnum<class "_Controller.lvclass">)  [unwired: 10 in, 1 out]
        n151 = control-ref of="ABORT"() -> (w291:refnum<vi>)
        n152 = call "Xn.vi"("Position"=55000, "_Controller in"=w292) -> ("_Controller out"=w290:refnum<class "_Controller.lvclass">)  [unwired: 8 in, 1 out]
        n153 = call "WAIT 0.vi"("reference"=w291, "_Controller in"=w290) -> ("_Controller out"=w303:refnum<class "_Controller.lvclass">)  [unwired: 7 in, 2 out]
        n154 = call "Motor speed settings.vi"("reference (in)"=w303, "HSPD"=100 ("High Speed"), "LSPD"=100 ("Low Speed"), "ACC"=10 ("Acceleration Time")) -> ("reference (out)"=w308:refnum<class "_Controller.lvclass">)  [unwired: 10 in, 1 out]
        n155 = while {
          tunnel: w308 -> [w327]
          tunnel: [w321] -> w302
          tunnel: [w324] -> w312
          tunnel: [w323] -> w306
          stop <- w323 continue-if-true
          n156 = local read "Approaching"() -> (w328:bool)
          n157 = local read "ABORT"() -> (w324:bool)
          n158 = control-ref of="ABORT"() -> (w320:refnum<vi>)
          n159 = call "Xn.vi"("Position"=15, "_Controller in"=w327) -> ("_Controller out"=w322:refnum<class "_Controller.lvclass">)  [unwired: 8 in, 1 out]
          n160 = Not(x=w324) -> (.not. x?=w325:bool)
          n161 = And(x=w328, y=w325) -> (x .and. y?=w323:bool)
          n162 = call "WAIT 0.vi"("reference"=w320, "_Controller in"=w322) -> ("_Controller out"=w321:refnum<class "_Controller.lvclass">)  [unwired: 7 in, 2 out]
        }
        n163 = local write "Approaching"(w306) -> ()
        n164 = Select(t=Motor_states."Terminate", s=w312, f=Motor_states."Testing") -> (s? t:f=w313:T5)
      }
      frame "Testing" {
        n165 = local write "Testing"(TRUE ("Testing")) -> ()
        n166 = local read "x-Velocity [mm/s]"() -> (w351:i32)
        n167 = call "mm-s to pps.vi"("Numeric Control in"=w351) -> ("Numeric Control out"=w348:i32)  [unwired: 10 in]
        n168 = call "Motor speed settings.vi"("reference (in)"=w335, "HSPD"=1000, "LSPD"=1000, "ACC"=10) -> ("reference (out)"=w341:refnum<class "_Controller.lvclass">)  [unwired: 10 in, 1 out]
        n169 = call "Motor speed settings.vi"("reference (in)"=w333, "HSPD"=w348, "LSPD"=1000, "ACC"=250) -> ("reference (out)"=w338:refnum<class "_Controller.lvclass">)  [unwired: 10 in, 1 out]
        n170 = local read "Track length [mm]"() -> (w358:i32)
        n171 = local read "Wear cycles"() -> (w353:i32)
        n172 = call <instrlib>:"send_receive_command.vi"("reference (in)"=w338, "ASCII Command (in)"="PX=0") -> ("reference (out)"=w337:refnum<class "_Controller.lvclass">)  [unwired: 13 in, 4 out]
        n173 = call <instrlib>:"send_receive_command.vi"("reference (in)"=w341, "ASCII Command (in)"="PX=0") -> ("reference (out)"=w340:refnum<class "_Controller.lvclass">)  [unwired: 13 in, 4 out]
        n174 = Multiply(x=w358, y=800) -> (x*y=w356:i32)
        n175 = Multiply(x=w353, y=2) -> (x*y=w330:i32)
        n176 = while {
          tunnel: w340 -> [w371]
          tunnel: [w361] -> w334
          tunnel: w343 -> [w362]
          i -> [w369]
          stop <- w365 continue-if-true
          n177 = Dequeue Element(queue=w362) -> (element=w363:i32, error out=w364:errorcluster)  [unwired: 2 in, 2 out]
          "received P" <- w363
          n178 = call <vilib>:"Clear Errors.vi"("error in (no error)"=w364) -> ()  [unwired: 5 in, 2 out]
          n179 = call "Xn.vi"("Position"=w363, "_Controller in"=w371) -> ("_Controller out"=w370:refnum<class "_Controller.lvclass">)  [unwired: 8 in, 1 out]
          n180 = local read "Testing"() -> (w366:bool)
          n181 = local read "ABORT"() -> (w368:bool)
          n182 = control-ref of="ABORT"() -> (w360:refnum<vi>)
          n183 = call "WAIT 0.vi"("reference"=w360, "_Controller in"=w370) -> ("_Controller out"=w361:refnum<class "_Controller.lvclass">)  [unwired: 7 in, 2 out]
          n184 = Not(x=w368) -> (.not. x?=w367:bool)
          n185 = And(x=w366, y=w367) -> (x .and. y?=w365:bool)
          "Correction loop" <- w369
        }
        n186 = Negate(x=w356) -> (-x=w355:i32)
        n187 = for {
          N: w330 -> [w376]
          tunnel: w337 -> [w383]
          tunnel: [w379] -> w332
          tunnel: w356 -> [w382]
          tunnel: w355 -> [w381]
          tunnel: [FALSE ("Testing")] -> w354
          i -> [w375]
          stop <- w377 stop-if-true
          n188 = local write "Test Progress"(w375) -> ()
          n189 = Quotient & Remainder(x=w375, y=2) -> (x-y*floor(x/y)=w385:i32)  [unwired: 1 out]
          n190 = Equal To 0?(x=w385) -> (x = 0?=w384:bool)
          n191 = case shown="False" w384 {
            tunnel: w383 -> [w390 w393]
            tunnel: [w389 w392] -> w380
            tunnel: w382 -> [_ w391]
            tunnel: w381 -> [w388 _]
            frame False {
              n192 = call "Xn.vi"("Position"=w388, "_Controller in"=w390) -> ("_Controller out"=w389:refnum<class "_Controller.lvclass">)  [unwired: 8 in, 1 out]
            }
            frame True {
              n193 = call "Xn.vi"("Position"=w391, "_Controller in"=w393) -> ("_Controller out"=w392:refnum<class "_Controller.lvclass">)  [unwired: 8 in, 1 out]
            }
          }
          n194 = Subtract(x=w376, y=w375) -> (x-y=w374:i32)
          n195 = control-ref of="ABORT"() -> (w378:refnum<vi>)
          n196 = Quotient & Remainder(x=w374, y=2) -> (floor(x/y)=w372:i32)  [unwired: 1 out]
          n197 = property on="Cycles left" class="DigNum (strict)"("Val(Sgnl)"=w372) -> ()  [unwired: 2 in, 2 out]
          n198 = call "WAIT 0.vi"("reference"=w378, "_Controller in"=w380) -> ("_Controller out"=w379:refnum<class "_Controller.lvclass">, "ABORT"=w377:bool)  [unwired: 7 in, 1 out]
        }
        n199 = Decrement(x=w330) -> (x-1=w329:i32)
        n200 = property on="Test Progress" class="Slide (strict)"("Scale.Maximum"=w329) -> ()  [unwired: 2 in, 2 out]
        n201 = local write "Testing"(w354) -> ()
      }
      frame "Terminate" {
        n202 = control-ref of="ABORT"() -> (w396:refnum<vi>)
        n203 = control-ref of="ABORT"() -> (w397:refnum<vi>)
        n204 = Unbundle(w406) -> ("queue out"=w405:refnum<queue>, "queue out"=w404:refnum<queue>, "queue out"=w403:refnum<queue>)
        n205 = case shown="False" FALSE {
          tunnel: w401 -> [w419 w436]
          tunnel: [w418 w433] -> w398
          frame False {
            n206 = call "Motor speed settings.vi"("reference (in)"=w419, "HSPD"=22000, "LSPD"=1000, "ACC"=500) -> ("reference (out)"=w424:refnum<class "_Controller.lvclass">)  [unwired: 10 in, 1 out]
            n207 = Negate(x=600 ("Position")) -> (-x=w425:i32)
            n208 = call "Xn.vi"("Position"=w425, "_Controller in"=w424) -> ("_Controller out"=w426:refnum<class "_Controller.lvclass">)  [unwired: 8 in, 1 out]
            n209 = control-ref of="ABORT"() -> (w417:refnum<vi>)
            n210 = call "WAIT 0.vi"("reference"=w417, "_Controller in"=w426) -> ("_Controller out"=w418:refnum<class "_Controller.lvclass">)  [unwired: 7 in, 2 out]
          }
          frame True {
            n211 = call "Motor speed settings.vi"("reference (in)"=w436, "HSPD"=22000, "LSPD"=1000, "ACC"=500) -> ("reference (out)"=w430:refnum<class "_Controller.lvclass">)  [unwired: 10 in, 1 out]
            n212 = Negate(x=80000 ("Position")) -> (-x=w431:i32)
            n213 = call "Xn.vi"("Position"=w431, "_Controller in"=w430) -> ("_Controller out"=w434:refnum<class "_Controller.lvclass">)  [unwired: 8 in, 1 out]
            n214 = control-ref of="ABORT"() -> (w435:refnum<vi>)
            n215 = call "WAIT 0.vi"("reference"=w435, "_Controller in"=w434) -> ("_Controller out"=w433:refnum<class "_Controller.lvclass">)  [unwired: 7 in, 2 out]
          }
        }
        n216 = call "WAIT 0.vi"("reference"=w396, "_Controller in"=w399) -> ("_Controller out"=w409:refnum<class "_Controller.lvclass">)  [unwired: 7 in, 2 out]
        n217 = call "WAIT 0.vi"("reference"=w397, "_Controller in"=w400) -> ("_Controller out"=w414:refnum<class "_Controller.lvclass">)  [unwired: 7 in, 2 out]
        n218 = Release Queue(queue=w402) -> ()  [unwired: 2 in, 3 out]
        n219 = Release Queue(queue=w403) -> ()  [unwired: 2 in, 3 out]
        n220 = call <instrlib>:"send_receive_command.vi"("reference (in)"=w409, "ASCII Command (in)"="SR0=1") -> ("reference (out)"=w410:refnum<class "_Controller.lvclass">)  [unwired: 13 in, 4 out]
        n221 = Release Queue(queue=w404) -> ()  [unwired: 2 in, 3 out]
        n222 = call <instrlib>:"send_receive_command.vi"("reference (in)"=w414, "ASCII Command (in)"="SR0=1") -> ("reference (out)"=w413:refnum<class "_Controller.lvclass">)  [unwired: 13 in, 4 out]
        n223 = Release Queue(queue=w405) -> ()  [unwired: 2 in, 3 out]
        n224 = call <instrlib>:"close_connection.vi"("reference (in)"=w410) -> ()  [unwired: 17 in, 2 out]
        n225 = call <instrlib>:"close_connection.vi"("reference (in)"=w413) -> ()  [unwired: 17 in, 2 out]
        n226 = call <instrlib>:"send_receive_command.vi"("reference (in)"=w398, "ASCII Command (in)"="SR0=1") -> ("reference (out)"=w415:refnum<class "_Controller.lvclass">)  [unwired: 13 in, 4 out]
        n227 = call <instrlib>:"close_connection.vi"("reference (in)"=w415) -> ("error out"=w395:errorcluster)  [unwired: 17 in, 1 out]
        n228 = local read "ABORT"() -> (w408:bool)
        n229 = case shown="True" w408 {
          tunnel: [w437 w438] -> w407
          tunnel: w395 -> [_ _]
          frame False {
            w437 = TRUE ("Value (Signaling)")
            n230 = property on="ABORT" class="Bool (strict)"("Val(Sgnl)"=w437) -> ()  [unwired: 2 in, 2 out]
            n231 = local write "Completed"(w437) -> ()
          }
          frame True {
            w438 = TRUE ("Value (Signaling)")
            n232 = local write "Aborted"(w438) -> ()
          }
        }
      }
    }
  }
  n233 = Format Into String(Queue_names."x-axis ref queue" ("Enum")) -> (resulting string=w16:string)  [unwired: 3 in, 1 out]
  n234 = Format Into String(Queue_names."y-axis ref queue" ("Enum")) -> (resulting string=w17:string)  [unwired: 3 in, 1 out]
  n235 = Format Into String(Queue_names."z-axis ref queue" ("Enum")) -> (resulting string=w15:string)  [unwired: 3 in, 1 out]
  n236 = Obtain Queue(name (unnamed)=w15, element data type=w1) -> (queue out=w7:refnum<queue>, error out=w6:errorcluster)  [unwired: 3 in, 1 out]
  n237 = Obtain Queue(name (unnamed)=w16, element data type=w1) -> (queue out=w9:refnum<queue>, error out=w8:errorcluster)  [unwired: 3 in, 1 out]
  n238 = Obtain Queue(name (unnamed)=w17, element data type=w1) -> (queue out=w11:refnum<queue>, error out=w10:errorcluster)  [unwired: 3 in, 1 out]
  n239 = while "Manual Control Enabling Loop" {
    tunnel: w11 -> [w454]
    tunnel: w10 -> [w453]
    tunnel: w9 -> [w452]
    tunnel: w8 -> [w451]
    tunnel: w7 -> [w450]
    tunnel: w6 -> [w449]
    tunnel: [w444] -> w5
    tunnel: [w443] -> w4
    tunnel: [w442] -> w3
    stop <- w455 stop-if-true
    n240 = Preview Queue Element(queue=w450, error in (no error)=w449) -> (queue out=w448:refnum<queue>, element=w441:refnum<class "_Controller.lvclass">)  [unwired: 1 in, 2 out]
    n241 = Preview Queue Element(queue=w452, error in (no error)=w451) -> (queue out=w447:refnum<queue>, element=w440:refnum<class "_Controller.lvclass">)  [unwired: 1 in, 2 out]
    n242 = Preview Queue Element(queue=w454, error in (no error)=w453) -> (queue out=w446:refnum<queue>, element=w439:refnum<class "_Controller.lvclass">)  [unwired: 1 in, 2 out]
    n243 = Bundle("queue out"=w448, "queue out"=w447, "queue out"=w446) -> (w445:T12)  [unwired: 1 in]
    n244 = event shown="[4] \"Left\": Value Change" {
      selector: _ -> [_ _ _ _ _ _ _ _ _ _]
      dyn-events: _ -> [_ _ _ _ _ _ _ _ _ _]
      timeout: _ -> [_ _ _ _ _ _ _ _ _ _]
      tunnel: w441 -> [_ _ w494 w505 _ _ _ _ _ _]
      tunnel: w440 -> [_ _ _ _ w516 w527 _ _ _ _]
      tunnel: w439 -> [_ _ _ _ _ _ w538 w549 _ _]
      tunnel: [_ _ _ _ _ _ _ _ _ w564] -> w455
      event Timeout {
        n245 = event-data() -> ()  [unwired: 1 in, 3 out]
      }
      event Key Down; Key Up {
        n246 = event-data() -> ("Type"=w457:T14, "ScanCode"=w458:i16)  [unwired: 1 in, 2 out]
        n247 = property on="Manual control" class="Bool (strict)"() -> ("Value"=w456:bool)  [unwired: 2 in, 2 out]
        n248 = case shown="True" w456 {
          tunnel: w458 -> [_ w460]
          tunnel: w457 -> [_ w459]
          frame False {
          }
          frame True {
            n249 = case shown="20" w460 {
              tunnel: w459 -> [_ w462 w467 w472 w477 w482 w487 w491]
              frame 0, Default {
              }
              frame 72 {
                # "Up"
                n250 = local read "Down"() -> (w461:bool)
                n251 = case shown="False" w461 {
                  tunnel: w462 -> [w463 _]
                  frame False {
                    n252 = case shown="\"Key Down\"" w463 {
                      frame "Null", Default {
                      }
                      frame "Key Down" {
                        n253 = property on="Up" class="Bool (strict)"("Val(Sgnl)"=TRUE) -> ()  [unwired: 2 in, 2 out]
                      }
                      frame "Key Up" {
                        n254 = property on="Up" class="Bool (strict)"("Val(Sgnl)"=FALSE) -> ()  [unwired: 2 in, 2 out]
                      }
                    }
                  }
                  frame True {
                  }
                }
              }
              frame 80 {
                # "Down"
                n255 = local read "Up"() -> (w466:bool)
                n256 = case shown="False" w466 {
                  tunnel: w467 -> [w468 _]
                  frame False {
                    n257 = case shown="\"Key Up\"" w468 {
                      frame "Null", Default {
                      }
                      frame "Key Down" {
                        n258 = property on="Down" class="Bool (strict)"("Val(Sgnl)"=TRUE) -> ()  [unwired: 2 in, 2 out]
                      }
                      frame "Key Up" {
                        n259 = property on="Down" class="Bool (strict)"("Val(Sgnl)"=FALSE) -> ()  [unwired: 2 in, 2 out]
                      }
                    }
                  }
                  frame True {
                  }
                }
              }
              frame 75 {
                # "Left"
                n260 = local read "Right"() -> (w471:bool)
                n261 = case shown="False" w471 {
                  tunnel: w472 -> [w473 _]
                  frame False {
                    n262 = case shown="\"Key Up\"" w473 {
                      frame "Null", Default {
                      }
                      frame "Key Down" {
                        n263 = property on="Left" class="Bool (strict)"("Val(Sgnl)"=TRUE) -> ()  [unwired: 2 in, 2 out]
                      }
                      frame "Key Up" {
                        n264 = property on="Left" class="Bool (strict)"("Val(Sgnl)"=FALSE) -> ()  [unwired: 2 in, 2 out]
                      }
                    }
                  }
                  frame True {
                  }
                }
              }
              frame 77 {
                # "Right"
                n265 = local read "Left"() -> (w476:bool)
                n266 = case shown="False" w476 {
                  tunnel: w477 -> [w478 _]
                  frame False {
                    n267 = case shown="\"Key Up\"" w478 {
                      frame "Null", Default {
                      }
                      frame "Key Down" {
                        n268 = property on="Right" class="Bool (strict)"("Val(Sgnl)"=TRUE) -> ()  [unwired: 2 in, 2 out]
                      }
                      frame "Key Up" {
                        n269 = property on="Right" class="Bool (strict)"("Val(Sgnl)"=FALSE) -> ()  [unwired: 2 in, 2 out]
                      }
                    }
                  }
                  frame True {
                  }
                }
              }
              frame 24 {
                # "Out"
                n270 = local read "In"() -> (w481:bool)
                n271 = case shown="False" w481 {
                  tunnel: w482 -> [w483 _]
                  frame False {
                    n272 = case shown="\"Key Up\"" w483 {
                      frame "Null", Default {
                      }
                      frame "Key Down" {
                        n273 = property on="Out" class="Bool (strict)"("Val(Sgnl)"=TRUE) -> ()  [unwired: 2 in, 2 out]
                      }
                      frame "Key Up" {
                        n274 = property on="Out" class="Bool (strict)"("Val(Sgnl)"=FALSE) -> ()  [unwired: 2 in, 2 out]
                      }
                    }
                  }
                  frame True {
                  }
                }
              }
              frame 23 {
                # "In"
                n275 = local read "Out"() -> (w486:bool)
                n276 = case shown="False" w486 {
                  tunnel: w487 -> [w488 _]
                  frame False {
                    n277 = case shown="\"Key Up\"" w488 {
                      frame "Null", Default {
                      }
                      frame "Key Down" {
                        n278 = property on="In" class="Bool (strict)"("Val(Sgnl)"=TRUE) -> ()  [unwired: 2 in, 2 out]
                      }
                      frame "Key Up" {
                        n279 = property on="In" class="Bool (strict)"("Val(Sgnl)"=FALSE) -> ()  [unwired: 2 in, 2 out]
                      }
                    }
                  }
                  frame True {
                  }
                }
              }
              frame 20 {
                n280 = case shown="\"Key Down\"" w491 {
                  frame "Null", Default {
                  }
                  frame "Key Down" {
                    n281 = local write "TARE"(TRUE ("TARE")) -> ()
                  }
                }
              }
            }
          }
        }
      }
      event "Up": Value Change {
        n282 = event-data() -> ()  [unwired: 1 in, 1 out]
        n283 = property on="Manual control" class="Bool (strict)"() -> ("Value"=w493:bool)  [unwired: 2 in, 2 out]
        n284 = case shown="True" w493 {
          tunnel: w494 -> [_ w495]
          frame False {
          }
          frame True {
            n285 = local read "Up"() -> (w496:bool)
            n286 = case shown="True" w496 {
              tunnel: w495 -> [w500 w503]
              frame False {
                n287 = call <instrlib>:"send_receive_command.vi"("reference (in)"=w500, "ASCII Command (in)"="STOP") -> ("reference (out)"=w498:refnum<class "_Controller.lvclass">)  [unwired: 13 in, 4 out]
                n288 = property on="Down" class="Bool (strict)"("DisabledEnum"=T7."Enabled" ("Disabled")) -> ()  [unwired: 2 in, 2 out]
                n289 = call "WAITX.vi"("_Controller in"=w498) -> ()  [unwired: 8 in, 3 out]
              }
              frame True {
                n290 = call-dynamic "jogMotor.vi"("Controller in"=w503, "dir"=linear_direction."NEG (-)") -> ()  [unwired: 14 in, 4 out]
                n291 = property on="Down" class="Bool (strict)"("DisabledEnum"=T7."Disabled" ("Disabled")) -> ()  [unwired: 2 in, 2 out]
              }
            }
          }
        }
      }
      event "Down": Value Change {
        n292 = event-data() -> ()  [unwired: 1 in, 1 out]
        n293 = property on="Manual control" class="Bool (strict)"() -> ("Value"=w504:bool)  [unwired: 2 in, 2 out]
        n294 = case shown="True" w504 {
          tunnel: w505 -> [_ w507]
          frame False {
          }
          frame True {
            n295 = local read "Down"() -> (w506:bool)
            n296 = case shown="True" w506 {
              tunnel: w507 -> [w511 w514]
              frame False {
                n297 = call <instrlib>:"send_receive_command.vi"("reference (in)"=w511, "ASCII Command (in)"="STOP") -> ("reference (out)"=w509:refnum<class "_Controller.lvclass">)  [unwired: 13 in, 4 out]
                n298 = property on="Up" class="Bool (strict)"("DisabledEnum"=T7."Enabled" ("Disabled")) -> ()  [unwired: 2 in, 2 out]
                n299 = call "WAITX.vi"("_Controller in"=w509) -> ()  [unwired: 8 in, 3 out]
              }
              frame True {
                n300 = call-dynamic "jogMotor.vi"("Controller in"=w514, "dir"=linear_direction."POS (+)") -> ()  [unwired: 14 in, 4 out]
                n301 = property on="Up" class="Bool (strict)"("DisabledEnum"=T7."Disabled" ("Disabled")) -> ()  [unwired: 2 in, 2 out]
              }
            }
          }
        }
      }
      event "Left": Value Change {
        n302 = event-data() -> ()  [unwired: 1 in, 1 out]
        n303 = property on="Manual control" class="Bool (strict)"() -> ("Value"=w515:bool)  [unwired: 2 in, 2 out]
        n304 = case shown="True" w515 {
          tunnel: w516 -> [_ w518]
          frame False {
          }
          frame True {
            n305 = local read "Left"() -> (w517:bool)
            n306 = case shown="True" w517 {
              tunnel: w518 -> [w522 w525]
              frame False {
                n307 = call <instrlib>:"send_receive_command.vi"("reference (in)"=w522, "ASCII Command (in)"="STOP") -> ("reference (out)"=w520:refnum<class "_Controller.lvclass">)  [unwired: 13 in, 4 out]
                n308 = call "WAITX.vi"("_Controller in"=w520) -> ()  [unwired: 8 in, 3 out]
                n309 = property on="Right" class="Bool (strict)"("DisabledEnum"=T7."Enabled" ("Disabled")) -> ()  [unwired: 2 in, 2 out]
              }
              frame True {
                n310 = call-dynamic "jogMotor.vi"("Controller in"=w525, "dir"=linear_direction."NEG (-)") -> ()  [unwired: 14 in, 4 out]
                n311 = property on="Right" class="Bool (strict)"("DisabledEnum"=T7."Enabled" ("Disabled")) -> ()  [unwired: 2 in, 2 out]
              }
            }
          }
        }
      }
      event "Right": Value Change {
        n312 = event-data() -> ()  [unwired: 1 in, 1 out]
        n313 = property on="Manual control" class="Bool (strict)"() -> ("Value"=w526:bool)  [unwired: 2 in, 2 out]
        n314 = case shown="True" w526 {
          tunnel: w527 -> [_ w529]
          frame False {
          }
          frame True {
            n315 = local read "Right"() -> (w528:bool)
            n316 = case shown="False" w528 {
              tunnel: w529 -> [w533 w536]
              frame False {
                n317 = call <instrlib>:"send_receive_command.vi"("reference (in)"=w533, "ASCII Command (in)"="STOP") -> ("reference (out)"=w531:refnum<class "_Controller.lvclass">)  [unwired: 13 in, 4 out]
                n318 = call "WAITX.vi"("_Controller in"=w531) -> ()  [unwired: 8 in, 3 out]
                n319 = property on="Left" class="Bool (strict)"("DisabledEnum"=T7."Enabled" ("Disabled")) -> ()  [unwired: 2 in, 2 out]
              }
              frame True {
                n320 = call-dynamic "jogMotor.vi"("Controller in"=w536, "dir"=linear_direction."POS (+)") -> ()  [unwired: 14 in, 4 out]
                n321 = property on="Left" class="Bool (strict)"("DisabledEnum"=T7."Disabled" ("Disabled")) -> ()  [unwired: 2 in, 2 out]
              }
            }
          }
        }
      }
      event "Out": Value Change {
        n322 = event-data() -> ()  [unwired: 1 in, 1 out]
        n323 = property on="Manual control" class="Bool (strict)"() -> ("Value"=w537:bool)  [unwired: 2 in, 2 out]
        n324 = case shown="True" w537 {
          tunnel: w538 -> [_ w540]
          frame False {
          }
          frame True {
            n325 = local read "Out"() -> (w539:bool)
            n326 = case shown="True" w539 {
              tunnel: w540 -> [w544 w547]
              frame False {
                n327 = call <instrlib>:"send_receive_command.vi"("reference (in)"=w544, "ASCII Command (in)"="STOP") -> ("reference (out)"=w542:refnum<class "_Controller.lvclass">)  [unwired: 13 in, 4 out]
                n328 = property on="In" class="Bool (strict)"("DisabledEnum"=T7."Enabled" ("Disabled")) -> ()  [unwired: 2 in, 2 out]
                n329 = call "WAITX.vi"("_Controller in"=w542) -> ()  [unwired: 8 in, 3 out]
              }
              frame True {
                n330 = call-dynamic "jogMotor.vi"("Controller in"=w547, "dir"=linear_direction."NEG (-)") -> ()  [unwired: 14 in, 4 out]
                n331 = property on="In" class="Bool (strict)"("DisabledEnum"=T7."Disabled" ("Disabled")) -> ()  [unwired: 2 in, 2 out]
              }
            }
          }
        }
      }
      event "In": Value Change {
        n332 = event-data() -> ()  [unwired: 1 in, 1 out]
        n333 = property on="Manual control" class="Bool (strict)"() -> ("Value"=w548:bool)  [unwired: 2 in, 2 out]
        n334 = case shown="True" w548 {
          tunnel: w549 -> [_ w551]
          frame False {
          }
          frame True {
            n335 = local read "In"() -> (w550:bool)
            n336 = case shown="True" w550 {
              tunnel: w551 -> [w555 w556]
              frame False {
                n337 = call <instrlib>:"send_receive_command.vi"("reference (in)"=w555, "ASCII Command (in)"="STOP") -> ("reference (out)"=w553:refnum<class "_Controller.lvclass">)  [unwired: 13 in, 4 out]
                n338 = call "WAITX.vi"("_Controller in"=w553) -> ()  [unwired: 8 in, 3 out]
                n339 = property on="Out" class="Bool (strict)"("DisabledEnum"=T7."Enabled" ("Disabled")) -> ()  [unwired: 2 in, 2 out]
              }
              frame True {
                n340 = call-dynamic "jogMotor.vi"("Controller in"=w556, "dir"=linear_direction."POS (+)") -> ()  [unwired: 14 in, 4 out]
                n341 = property on="Out" class="Bool (strict)"("DisabledEnum"=T7."Disabled" ("Disabled")) -> ()  [unwired: 2 in, 2 out]
              }
            }
          }
        }
      }
      event "Approach": Value Change {
        n342 = event-data() -> ()  [unwired: 1 in, 1 out]
        n343 = local read "Manual control"() -> (w559:bool)
        n344 = case shown="True" w559 {
          frame False {
          }
          frame True {
            n345 = local read "Approach"() -> (w560:bool)
            n346 = case shown="True" w560 {
              frame False {
              }
              frame True {
                n347 = flat-sequence {
                  tunnel: [FALSE ("Approach")] -> w561
                  frame #0 {
                    n348 = Wait Until Next ms Multiple(millisecond multiple=u32 300) -> ()  [unwired: 1 out]
                  }
                }
                n349 = local write "Approach"(w561) -> ()
              }
            }
          }
        }
      }
      event "ABORT": Value Change {
        n350 = event-data() -> ()  [unwired: 1 in, 1 out]
        n351 = local read "ABORT"() -> (w565:bool)
        n352 = case shown="False" w565 {
          tunnel: [FALSE TRUE] -> w564
          frame False {
          }
          frame True {
          }
        }
      }
    }
    n353 = Unbundle(w445) -> ("queue out"=w444:refnum<queue>, "queue out"=w443:refnum<queue>, "queue out"=w442:refnum<queue>)
  }
  n354 = Release Queue(queue=w5) -> ()  [unwired: 2 in, 3 out]
  n355 = Release Queue(queue=w4) -> ()  [unwired: 2 in, 3 out]
  n356 = Release Queue(queue=w3) -> ()  [unwired: 2 in, 3 out]
  n357 = while "Logic Loop" {
    shift-right: [w573] -> _
    shift-left: Logic_states."Initialize" ("Enum") -> [w574]
    shift-right: [w571] -> _
    shift-left: _ -> [w570]
    shift-right: [w569] -> _
    shift-left: _ -> [w568]
    stop <- w572 stop-if-true
    n358 = case shown="\"Initialize\", Default" w574 {
      tunnel: [w579 Logic_states."Terminate" ("Enum") _] -> w573
      tunnel: [_ _ TRUE] -> w572
      tunnel: [w588 w652 _] -> w571
      tunnel: w570 -> [_ w652 w738]
      tunnel: [w576 _ _] -> w569
      tunnel: w568 -> [_ w622 _]
      frame "Initialize", Default {
        n359 = call <vilib>:"Check if File or Folder Exists.vi"("path"="Save file name") -> ("file or folder exists?"=w586:bool, "dup path"=w585:path)  [unwired: 8 in, 1 out]
        n360 = case shown="True" w586 {
          tunnel: w585 -> [w610 w613]
          tunnel: [TRUE ("T button?") w618] -> w583
          tunnel: [w610 w613] -> w584
          tunnel: [FALSE w617] -> w580
          frame False {
          }
          frame True {
            n361 = Strip Path(path=w613) -> (name=w612:string)  [unwired: 1 out]
            n362 = Concatenate Strings("Warning!\nThis File already exists: " ("message"), "\r", w612) -> (w614:string)
            n363 = Two Button Dialog(message=w614, 1:"Abort" ("F button name (\"Cancel\")"), 2:"Overwrite" ("T button name (\"OK\")")) -> (T button?=w618:bool)
            n364 = Not(x=w618) -> (.not. x?=w617:bool)
            n365 = property on="ABORT" class="Bool (strict)"("Val(Sgnl)"=w617) -> ()  [unwired: 2 in, 2 out]
          }
        }
        n366 = case shown="True" w583 {
          tunnel: w584 -> [_ w608]
          tunnel: [_ w593] -> w576
          frame False {
          }
          frame True {
            n367 = local read "Sampling frequency (rate)"() -> (w602:T3)
            n368 = local read "Track length [mm]"() -> (w600:i32)
            n369 = local read "x-Velocity [mm/s]"() -> (w601:i32)
            n370 = local read "Wear cycles"() -> (w599:i32)
            n371 = Number To Decimal String(number=w602) -> (decimal integer string=w598:string)  [unwired: 1 in]
            n372 = Number To Decimal String(number=w601) -> (decimal integer string=w597:string)  [unwired: 1 in]
            n373 = Number To Decimal String(number=w600) -> (decimal integer string=w596:string)  [unwired: 1 in]
            n374 = Number To Decimal String(number=w599) -> (decimal integer string=w595:string)  [unwired: 1 in]
            n375 = Build Array("Sampling fequency [Hz]:", w598, "x-velocity [mm/s]: ", w597, "Track length [mm]:", w596, "Cycles:", w595) -> (w594:string[])
            n376 = call-poly <vilib>:"Write Delimited Spreadsheet.vi"("file path (dialog if empty)"=w608, "1D data"=w594) -> ("new file path (Not A Path if cancelled)"=w607:path)  [unwired: 12 in, 1 out]
            n377 = call-poly <vilib>:"Write Delimited Spreadsheet.vi"("file path (dialog if empty)"=w607, "1D data"=string[] ["Fx", "Fy", "Fz", "Tx", "Ty", "Tz", "x-Position"], "append to file? (new file:F)"=TRUE) -> ("new file path (Not A Path if cancelled)"=w593:path)  [unwired: 11 in, 1 out]
          }
        }
        n378 = Format Into String(Queue_names."Cell queue name" ("Enum")) -> (resulting string=w577:string)  [unwired: 3 in, 1 out]
        n379 = Obtain Queue(name (unnamed)=w577, element data type=dbl[] []) -> (queue out=w589:refnum<queue>, error out=w587:errorcluster)  [unwired: 3 in, 1 out]
        n380 = Bundle("queue out"=w589, "error out"=w587) -> (w588:T8)  [unwired: 1 in]
        n381 = Select(t=Logic_states."Terminate" ("Enum"), s=w580, f=Logic_states."Process" ("Enum")) -> (s? t:f=w579:T6)
      }
      frame "Process" {
        n382 = Unbundle(w652) -> ("queue out"=w628:refnum<queue>, "error out"=w627:errorcluster)
        n383 = local read "Sampling frequency (rate)"() -> (w649:T3)
        n384 = while "Saving Data" {
          tunnel: w622 -> [w722]
          tunnel: w628 -> [w721]
          tunnel: w627 -> [w720]
          stop <- w728 stop-if-true
          w725 = u16 2 items=["x-load", "y-load", "z-load", "x-torque", "y-torque", "z-torque"]
          n385 = Flush Queue(queue=w721, error in (no error)=w720) -> (remaining elements=w726:cluster{dbl[]}[])  [unwired: 2 out]
          n386 = for {
            tunnel: w726 -> [w731] mode=indexing
            tunnel: [w730] -> w724 mode=indexing
            n387 = Unbundle(w731) -> (w730:dbl[])
          }
          n388 = call-poly <vilib>:"Write Delimited Spreadsheet.vi"("file path (dialog if empty)"=w722, "2D data"=w724, "append to file? (new file:F)"=TRUE) -> ()  [unwired: 11 in, 2 out]
          n389 = Index Array(array=w724, index (col)=w725) -> (element=w723:dbl[])  [unwired: 1 in]
          n390 = Negate(x=w723) -> (-x=→"Dequeued Data":dbl[])
          n391 = local read "ABORT"() -> (w728:bool)
        }
        n392 = Format Into String(Queue_names."x-axis ref queue" ("Enum")) -> (resulting string=w625:string)  [unwired: 3 in, 1 out]
        n393 = Obtain Queue(name (unnamed)=w625, element data type=refnum<class "_Controller.lvclass"> refnum ("reference (in)")) -> (queue out=w626:refnum<queue>)  [unwired: 3 in, 2 out]
        n394 = Preview Queue Element(queue=w626) -> (element=w623:refnum<class "_Controller.lvclass">)  [unwired: 2 in, 3 out]
        n395 = Less Or Equal?(x=w649, y=u16 50) -> (x <= y?=w651:bool)
        n396 = Reciprocal(x=w649) -> (1/x=w648:dbl)
        n397 = Multiply(x=1000.0, y=w648) -> (x*y=w646:dbl)
        n398 = Format Into String(Queue_names."Feedback" ("Enum")) -> (resulting string=w631:string)  [unwired: 3 in, 1 out]
        n399 = Select(t=w646, s=w651, f=10.0) -> (s? t:f=w637:dbl)
        n400 = Divide(x=w637, y=1000.0) -> (x/y=w638:dbl)
        n401 = Obtain Queue(max queue size (-1, unlimited)=1, name (unnamed)=w631, element data type=0) -> (queue out=w630:refnum<queue>)  [unwired: 2 in, 2 out]
        n402 = while "Time Left" {
          tunnel: w623 -> [w657]
          stop <- w653 stop-if-true
          n403 = call "Read-motor-settings.vi"("_Controller in"=w657) -> ("Cluster"=w658:cluster{"HSPD":i32, "LSPD":i32, "ACC":i32})  [unwired: 10 in]
          n404 = Unbundle By Name(w658) -> ("HSPD"=w656:i32, "LSPD"=w655:i32, "ACC"=w654:i32)
          n405 = event shown="[1] \"Cycles left\": Value Change" {
            selector: _ -> [_ _ _]
            dyn-events: _ -> [_ _ _]
            timeout: _ -> [_ _ _]
            tunnel: w656 -> [_ w664 _]
            tunnel: w655 -> [_ w663 _]
            tunnel: w654 -> [_ w662 _]
            tunnel: [_ _ w665] -> w653
            event Timeout {
              n406 = event-data() -> ()  [unwired: 1 in, 1 out]
            }
            event "Cycles left": Value Change {
              n407 = event-data() -> ()  [unwired: 1 in, 1 out]
              n408 = local read "Track length [mm]"() -> (w660:i32)
              n409 = local read "Cycles left"() -> (w661:i32)
              n410 = call "Time-left.vi"("HSPD [pps]"=w664, "LSPD [pps]"=w663, "ACC [ms]"=w662, "Cycles left"=w661, "Testing length [mm]"=w660) -> ("Minutes left"=w659:i32)  [unwired: 10 in]
              n411 = local write "Apprx. Min Left"(w659) -> ()
            }
            event "ABORT": Value Change {
              n412 = event-data() -> ()  [unwired: 1 in, 1 out]
              n413 = local read "ABORT"() -> (w666:bool)
              n414 = case shown="True" w666 {
                tunnel: [FALSE TRUE] -> w665
                frame False {
                }
                frame True {
                }
              }
            }
          }
        }
        n415 = Format Into String(Queue_names."to PID" ("Enum")) -> (resulting string=w642:string)  [unwired: 3 in, 1 out]
        n416 = Obtain Queue(max queue size (-1, unlimited)=1, name (unnamed)=w642, element data type=0.0) -> (queue out=w639:refnum<queue>)  [unwired: 2 in, 2 out]
        n417 = while "Averaging" {
          tunnel: w637 -> [w711]
          tunnel: w639 -> [w693]
          tunnel: [w691] -> w635
          stop <- w713 stop-if-true
          w710 = u16 0 items=["x-load", "y-load", "z-load", "x-torque", "y-torque", "z-torque"]
          w716 = u16 2 items=["x-load", "y-load", "z-load", "x-torque", "y-torque", "z-torque"]
          n418 = Wait (ms)(milliseconds to wait=w711) -> ()  [unwired: 1 out]
          n419 = local read "Current reading"() -> (w709:dbl[])
          n420 = Index Array(array=w709, index=w716) -> (element=w717:dbl)
          n421 = Index Array(array=w709, index=w710) -> (element=w707:dbl)
          n422 = Negate(x=w717) -> (-x=w714:dbl)
          n423 = local read "Averaging Level"() -> (w706:i32)
          n424 = control-ref of="Mean x"() -> (w708:refnum<vi>)
          n425 = local read "Averaging Level"() -> (w712:i32)
          n426 = control-ref of="Mean z"() -> (w715:refnum<vi>)
          n427 = call "Smoothing.vi"("Averaging Level"=w706, "Input reading"=w707, "Array in"=w708) -> ("mean"=w705:dbl)  [unwired: 8 in]
          "Smooth x" <- w705
          n428 = call "Smoothing.vi"("Averaging Level"=w712, "Input reading"=w714, "Array in"=w715) -> ("mean"=w692:dbl)  [unwired: 8 in]
          "Smooth z" <- w692
          "Actual Load" <- w692
          n429 = local read "Testing Load [N]"() -> (w703:dbl)
          n430 = local read "Manual control"() -> (w700:bool)
          n431 = Divide(x=w705, y=w692) -> (x/y=→"Estimated friction coefficient":dbl)
          n432 = local read "ABORT"() -> (w694:bool)
          n433 = Greater Or Equal?(x=w692, y=w703) -> (x >= y?=w702:bool)
          n434 = Not(x=w700) -> (.not. x?=w699:bool)
          n435 = And(x=w702, y=w699) -> (x .and. y?=w701:bool)
          n436 = Greater?(x=w692, y=33.0) -> (0:w697:bool)
          n437 = Or(x=w701, y=w694) -> (x .or. y?=w695:bool)
          n438 = And(x=w697, y=w699) -> (x .and. y?=w696:bool)
          n439 = case shown="True" w696 {
            frame False {
            }
            frame True {
              n440 = property on="ABORT" class="Bool (strict)"("Val(Sgnl)"=TRUE ("Value (Signaling)")) -> ()  [unwired: 2 in, 2 out]
            }
          }
          n441 = case shown="True" w695 {
            frame False {
            }
            frame True {
              n442 = local write "Approaching"(FALSE ("Approaching")) -> ()
            }
          }
          n443 = Lossy Enqueue Element(queue=w693, element=w692) -> (queue out=w691:refnum<queue>)  [unwired: 1 in, 3 out]
          n444 = local read "ABORT"() -> (w713:bool)
        }
        n445 = while "PID" {
          tunnel: w638 -> [w675]
          tunnel: w639 -> [w672]
          tunnel: w630 -> [w671]
          tunnel: [w670] -> w629
          i -> [w673]
          stop <- w674 stop-if-true
          n446 = local read "Testing"() -> (w669:bool)
          n447 = case shown="True" w669 {
            tunnel: w675 -> [_ _]
            tunnel: w672 -> [_ w689]
            tunnel: w671 -> [w677 w685]
            tunnel: [w677 w684] -> w670
            frame False {
              n448 = Wait (ms)(milliseconds to wait=u32 250) -> ()  [unwired: 1 out]
            }
            frame True {
              n449 = Dequeue Element(queue=w689) -> (element=w681:dbl, error out=w686:errorcluster)  [unwired: 2 in, 2 out]
              n450 = call <vilib>:"Clear Errors.vi"("error in (no error)"=w686) -> ()  [unwired: 5 in, 2 out]
              n451 = local read "Testing Load [N]"() -> (w682:dbl)
              n452 = call-poly <vilib>:"PID.vi"("output range"="output range", "PID gains"="PID gains", "process variable"=w681, "setpoint"=w682) -> ("dt out (s)"=→"dt out (s)":dbl, "output"=w688:dbl)  [unwired: 6 in]
              "Correction [N]" <- w688
              n453 = Quotient & Remainder(x=w688, y=0.015) -> (floor(x/y)=w680:dbl)  [unwired: 1 out]
              "correction [p]" <- w680
              n454 = To Long Integer(number=w680) -> (32bit integer=w683:i32)
              n455 = Lossy Enqueue Element(queue=w685, element=w683) -> (queue out=w684:refnum<queue>)  [unwired: 1 in, 3 out]
            }
          }
          n456 = local read "ABORT"() -> (w674:bool)
          "to PID" <- w673
        }
        n457 = Release Queue(queue=w629) -> ()  [unwired: 2 in, 3 out]
        n458 = Release Queue(queue=w635) -> ()  [unwired: 2 in, 3 out]
      }
      frame "Terminate" {
        n459 = Initialize Array(0.0 ("element")) -> (w734:dbl[])  [unwired: 1 in]
        n460 = Initialize Array(0.0 ("element")) -> (w735:dbl[])  [unwired: 1 in]
        n461 = Unbundle(w738) -> ("queue out"=w737:refnum<queue>, "error out"=w736:errorcluster)
        n462 = local write "Mean z"(w734) -> ()
        n463 = local write "Mean x"(w735) -> ()
        n464 = Release Queue(queue=w737, error in (no error)=w736) -> ()  [unwired: 1 in, 3 out]
      }
    }
  }
  "x-position" <- 0 ("x-position")
